vi "Generator.TestLauncher.vi"() -> ()   [LabVIEW 2016, in "Generator.lvclass"]
uses:
  Generator.lvclass
  <vilib>/JKI/JKI SMO/SMO/Typedefs/SMOState --Enum.ctl
  Typedefs/PrivateEvents--Generator.configGenerator.ctl
  Typedefs/PrivateEvents--Generator.resetGenerator.ctl
  Typedefs/PrivateEvents--Generator.configSampling.ctl
  C:/Program Files (x86)/National Instruments/LabVIEW 2016/vi.lib/JKI/JKI SMO/SMO/SMO.lvclass
  <vilib>/JKI/JKI SMO/SMO/SMO.lvclass
panel:
  out "Waveform Graph":waveform(dbl)[](graph)
  in  "configSampling":T1
  in  "resetGenerator":T2
  in  "configGenerator":T3
  in  "get new waveform":bool
  out "SMO State":T4
  out "error out":errorcluster
  in  "Stop":bool
  # "Generator SMO Test Launcher"
  # "For instructions on how to use the JKI State Machine Objects, examples and video tutorials, visit:\nhttp://jki.net/state-machine-objects/\n\nJKI State Machine Objects™\nhttp://jki.net/state-machine-objects/\nCopyright (C) 2005-2015, JKI <info@jki.net>\nALL RIGHTS RESERVED"
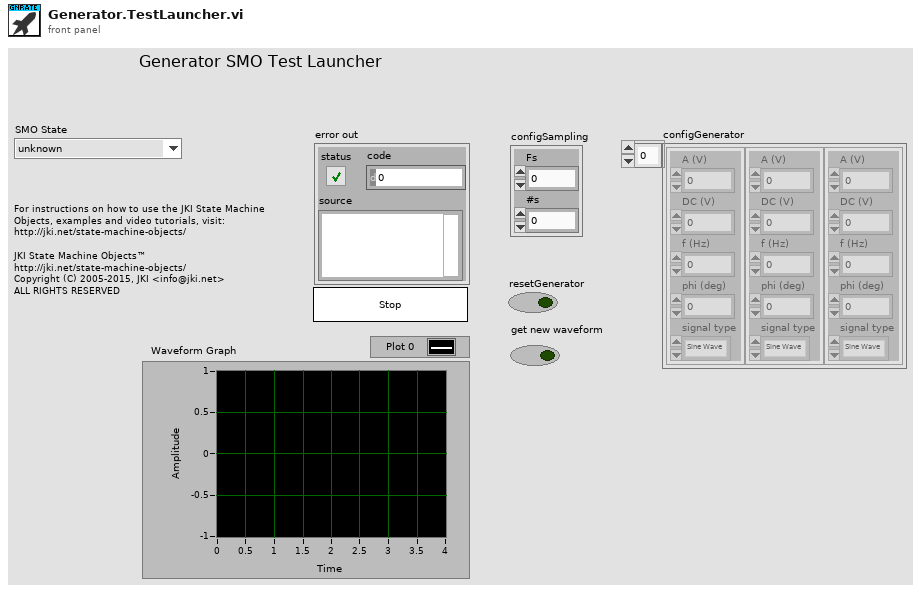
[diagram p1: front panel]
types:
  T1 = typedef "Generator.lvclass/PrivateEvents--Generator.configSampling.ctl" = cluster{"Fs":dbl, "#s":dbl}
  T2 = typedef "Generator.lvclass/PrivateEvents--Generator.resetGenerator.ctl" = bool
  T3 = typedef "Generator.lvclass/PrivateEvents--Generator.configGenerator.ctl" = cluster{"A (V)":dbl, "DC (V)":dbl, "f (Hz)":dbl, "phi (deg)":dbl, "signal type":enum16{"Sine Wave", "Triangle Wave", "Square Wave", "Sawtooth Wave"}}[]
  T4 = typedef "SMO.lvclass/SMOState --Enum.ctl" = enum16{"unknown", "Created", "Started", "Stopped"}
  T5 = typedef "SMO.lvclass/Public Events.ctl" = cluster{"Error":refnum<user-event>, "State":refnum<user-event>, "Reserve State":refnum<user-event>}
  T6 = typedef "Generator.lvclass/PublicEvents--Cluster.ctl" = cluster{"getGeneratorWaveforms":refnum<user-event>}
  T7 = cluster{"Event Registration Refnum":refnum<event-registration>}
  T8 = typedef "Generator.lvclass/PublicEvents--Generator.getGeneratorWaveforms.ctl" = waveform(dbl)[]
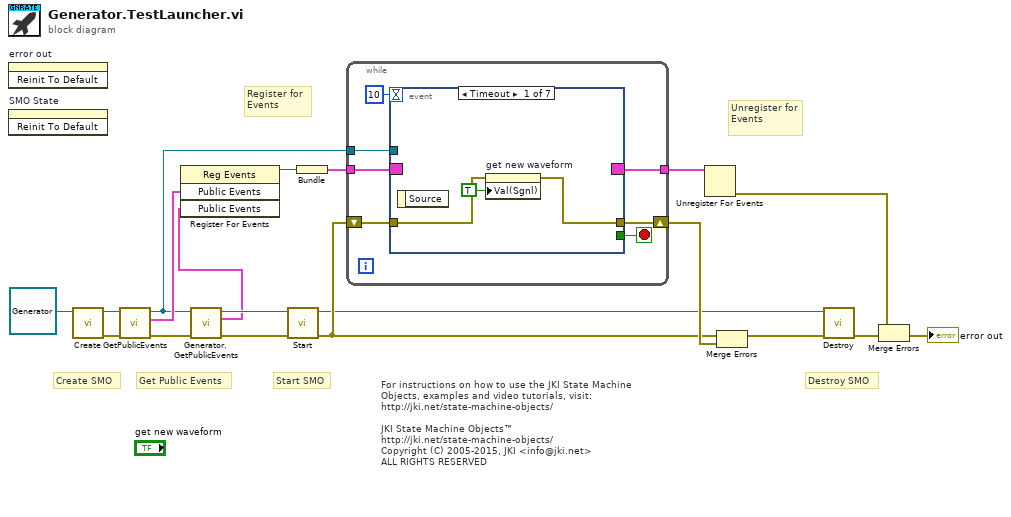
[diagram p0: block diagram]
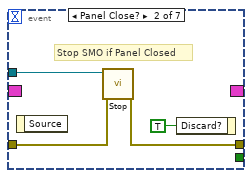
[diagram p2: hidden frame]
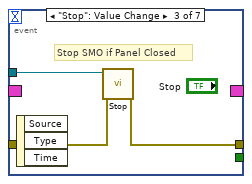
[diagram p3: hidden frame]
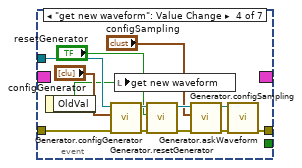
[diagram p4: hidden frame]
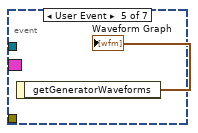
[diagram p5: hidden frame]
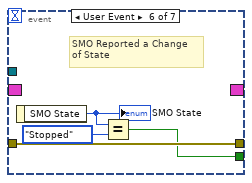
[diagram p6: hidden frame]
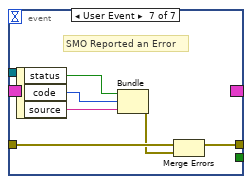
[diagram p7: hidden frame]
diagram:
  # "For instructions on how to use the JKI State Machine Objects, examples and video tutorials, visit:\nhttp://jki.net/state-machine-objects/\n\nJKI State Machine Objects™\nhttp://jki.net/state-machine-objects/\nCopyright (C) 2005-2015, JKI <info@jki.net>\nALL RIGHTS RESERVED"
  # "Get Public Events"
  # "Start SMO"
  # "Destroy SMO"
  # "Create SMO"
  # "Unregister for Events"
  # "Register for Events"
  n1 = invoke on="error out" class="Clust (strict)" method="Reinit To Default"() -> ()  [unwired: 3 in, 3 out]
  n2 = invoke on="SMO State" class="Enum (strict)" method="Reinit To Default"() -> ()  [unwired: 3 in, 3 out]
  n3 = call <vilib>:"Create.vi"("SMO"=refnum<class "Generator.lvclass"> refnum ("SMO.Template.lvclass")) -> ("error out"=w8:errorcluster, "SMO out"=w9:refnum<class "Generator.lvclass">)  [unwired: 8 in, 1 out]
  n4 = call <vilib>:"GetPublicEvents.vi"("error in (no error)"=w8, "SMO"=w9) -> ("error out"=w5:errorcluster, "Public Events"=w7:T5, "SMO out"=w4:refnum<class "Generator.lvclass">)  [unwired: 7 in]
  n5 = call "Generator.GetPublicEvents.vi"("error in (no error)"=w5, "Generator"=w4) -> ("error out"=w2:errorcluster, "Public Events"=w1:T6, "Generator out"=w3:refnum<class "Generator.lvclass">)  [unwired: 7 in]
  n6 = register-events(w7, w1) -> (reference out=w6:refnum<event-registration>)  [unwired: 2 in, 1 out]
  n7 = call <vilib>:"Start.vi"("error in (no error)"=w2, "SMO"=w3) -> ("error out"=w12:errorcluster, "SMO out"=w10:refnum<class "Generator.lvclass">)  [unwired: 8 in]
  n8 = Bundle("Event Registration Refnum"=w6) -> (w18:T7)  [unwired: 1 in]
  n9 = while {
    shift-right: [w25] -> w17
    shift-left: w12 -> [w24]
    tunnel: w18 -> [w23]
    tunnel: [w22] -> w19
    tunnel: w4 -> [w21]
    stop <- w26 stop-if-true
    n10 = event shown="[0] Timeout" {
      selector: w23 -> [_ _ _ _ _ _ _]
      dyn-events: [_ _ _ _ _ _ _] -> w22
      timeout: 10 -> [_ _ _ _ _ _ _]
      tunnel: [_ _ _ _ _ w51 _] -> w26
      tunnel: w21 -> [_ w33 w36 w45 _ _ _]
      tunnel: [w28 w32 w35 w39 _ w54 w58] -> w25
      tunnel: w24 -> [w29 w31 w34 w49 _ w54 w56]
      event Timeout {
        n11 = event-data() -> ()  [unwired: 1 in, 1 out]
        n12 = property on="get new waveform" class="Bool (strict)"(error in=w29, "Val(Sgnl)"=TRUE ("Value (Signaling)")) -> (error out=w28:errorcluster)  [unwired: 1 in, 1 out]
      }
      event Panel Close? {
        # "Stop SMO if Panel Closed"
        n13 = event-data() -> ()  [unwired: 1 in, 1 out]
        n14 = call <vilib>:"Stop.vi"("error in (no error)"=w31, "SMO"=w33) -> ("error out"=w32:errorcluster)  [unwired: 8 in, 1 out]
        n15 = event-data("Discard?"=TRUE ("OK")) -> ()  [unwired: 1 in, 1 out]
      }
      event "Stop": Value Change {
        # "Stop SMO if Panel Closed"
        n16 = event-data() -> ()  [unwired: 1 in, 3 out]
        n17 = call <vilib>:"Stop.vi"("error in (no error)"=w34, "SMO"=w36) -> ("error out"=w35:errorcluster)  [unwired: 8 in, 1 out]
      }
      event "get new waveform": Value Change {
        n18 = event-data() -> ("OldVal"=w37:bool)  [unwired: 1 in]
        n19 = call "Generator.configGenerator.vi"("error in (no error)"=w49, "configGenerator"="configGenerator", "Generator"=w45) -> ("error out"=w48:errorcluster, "Generator out"=w44:refnum<class "Generator.lvclass">)  [unwired: 7 in]
        n20 = local write "get new waveform"(w37) -> ()
        n21 = call "Generator.resetGenerator.vi"("error in (no error)"=w48, "resetGenerator"="resetGenerator", "Generator"=w44) -> ("error out"=w47:errorcluster, "Generator out"=w43:refnum<class "Generator.lvclass">)  [unwired: 7 in]
        n22 = call "Generator.configSampling.vi"("error in (no error)"=w47, "configSampling"="configSampling", "Generator"=w43) -> ("error out"=w40:errorcluster, "Generator out"=w38:refnum<class "Generator.lvclass">)  [unwired: 7 in]
        n23 = call "Generator.askWaveform.vi"("error in (no error)"=w40, "Generator"=w38) -> ("error out"=w39:errorcluster)  [unwired: 8 in, 1 out]
      }
      event User Event {
        n24 = event-data() -> ("getGeneratorWaveforms"=→"Waveform Graph":T8)  [unwired: 1 in]
      }
      event User Event {
        # "SMO Reported a Change\nof State"
        n25 = event-data() -> ("SMO State"=w53:T4)  [unwired: 1 in]
        "SMO State" <- w53
        n26 = Equal?(x=w53, y=SMOState_--Enum."Stopped") -> (x = y?=w51:bool)
      }
      event User Event {
        # "SMO Reported an Error"
        n27 = event-data() -> ("status"=w57:bool, "code"=w60:i32, "source"=w59:string)  [unwired: 1 in]
        n28 = Bundle("status"=w57, "code"=w60, "source"=w59) -> (w55:errorcluster)  [unwired: 1 in]
        n29 = Merge Errors(w56, w55) -> (w58:errorcluster)
      }
    }
  }
  n30 = Unregister For Events(event registration refnum=w19) -> (error out=w16:errorcluster)  [unwired: 1 in]
  n31 = Merge Errors(w12, w17) -> (w11:errorcluster)
  n32 = call <vilib>:"Destroy.vi"("error in (no error)"=w11, "SMO"=w10) -> ("error out"=w14:errorcluster)  [unwired: 9 in]
  n33 = Merge Errors(w16, w14) -> (→"error out":errorcluster)
